vi "Count Coins - Image.vi"() -> ()   [LabVIEW 2022 SP3]
uses:
  Coin Analyser/Coin Analyser.lvclass
  Coin Analyser/Coins.ctl
panel:
  out "Features":cluster{"x":i32, "y":i32, "diameter":i32}[](array[cluster])
  out "Image":T1(plugin-control)
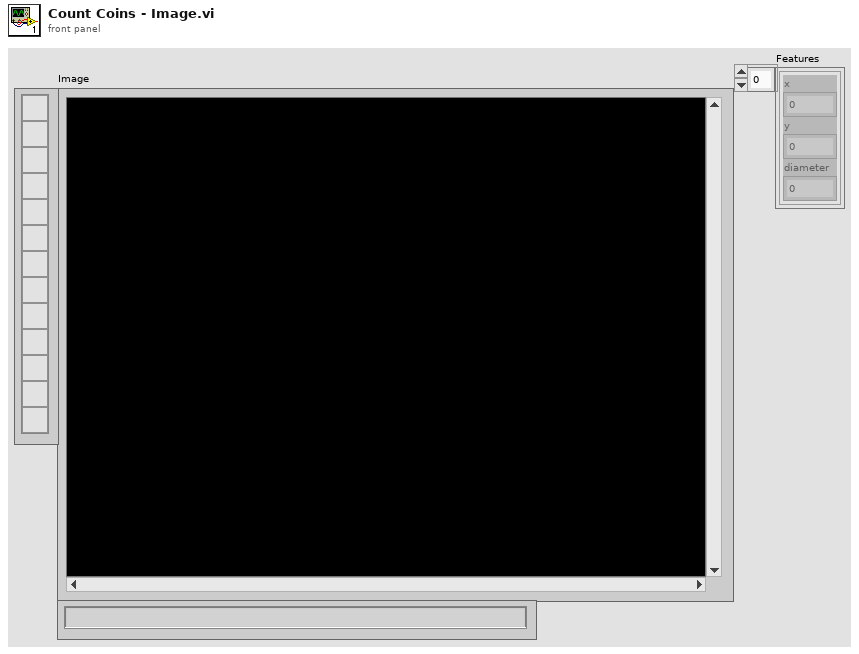
[diagram p1: front panel]
types:
  T1 = typedef "IMAQ Image.ctl" = refnum<image>
  T2 = typedef "Coin Analyser.lvclass/Coins.ctl" = cluster{"x":i32, "y":i32, "diameter":i32}
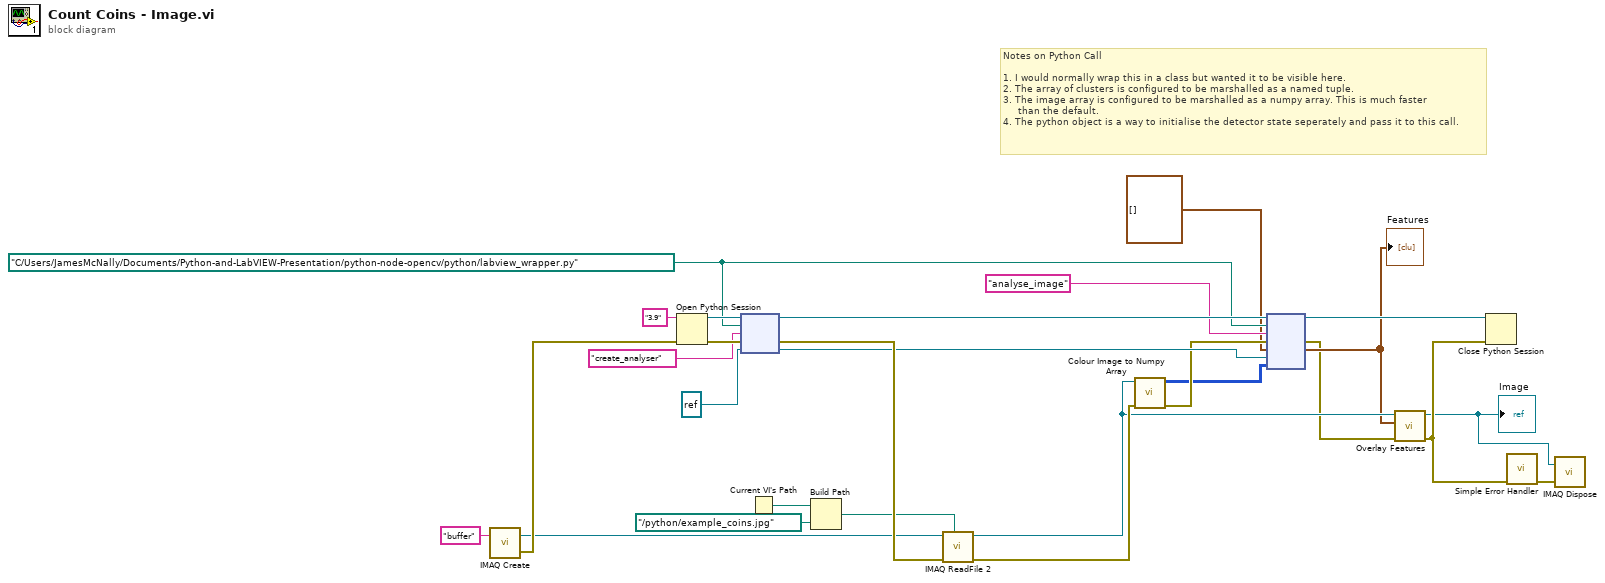
[diagram p0: block diagram]
diagram:
  w19 = path "C:/Users/JamesMcNally/Documents/Python-and-LabVIEW-Presentation/python-node-opencv/python/labview_wrapper.py" ("module path")
  # "Notes on Python Call\n\n1. I would normally wrap this in a class but wanted it to be visible here.\n2. The array of clusters is configured to be marshalled as a named tuple.\n3. The image array is configured to be marshalled as a numpy array. This is much faster\n     than the default.\n4. The python object is a way to initialise the detector state seperately and pass it to this call."
  n1 = call "IMAQ Create"("Image Name"="buffer") -> ("New Image"=w14:T1, "error out"=w15:errorcluster)  [unwired: 4 in]
  n2 = Open Python Session(python version="3.9" ("Python version"), 3:w15) -> (session out=w25:refnum<k35>, error out=w24:errorcluster)  [unwired: 1 in]
  n3 = node(w25, w19, "create_analyser" ("function name"), w24, refnum<k38> refnum ("Python Object Refnum")) -> (w21:refnum<k35>, w23:errorcluster, w18:refnum<k38>)  [unwired: 2 out]
  n4 = Current VI's Path() -> (path=w5:path)
  n5 = Build Path(base path=w5, name or relative path=path "../python/example_coins.jpg") -> (appended path=w3:path)
  n6 = call "IMAQ ReadFile 2"("File Path"=w3, "error in (no error)"=w23, "Image"=w14) -> ("error out"=w17:errorcluster, "Image Out"=w13:T1)  [unwired: 4 in, 3 out]
  n7 = call "Colour Image to Numpy Array.vi"("error in (no error)"=w17, "Refnum in"=w13) -> ("error out"=w10:errorcluster, "Array"=w7:u8[][][])  [unwired: 8 in]
  n8 = node(w21, w19, "analyse_image" ("function name"), w10, T2[] [], w18, w7) -> (w20:refnum<k35>, w6:errorcluster, w8:T2[])  [unwired: 2 in, 2 out]
  "Features" <- w8
  n9 = call "Overlay Features.vi"("error in (no error)"=w6, "Features"=w8, "Refnum in"=w13) -> ("Error Out"=w12:errorcluster, "Refnum out"=w1:T1)  [unwired: 7 in]
  "Image" <- w1
  n10 = Close Python Session(session in=w20, error in=w12) -> ()  [unwired: 1 out]
  n11 = call <vilib>:"Simple Error Handler.vi"("error in (no error)"=w12) -> ("error out"=w2:errorcluster)  [unwired: 4 in, 4 out]
  n12 = call "IMAQ Dispose"("Image"=w1, "error in (no error)"=w2) -> ()  [unwired: 4 in, 1 out]
